vi "GoHome.vi"(4 "Home fail":refnum<vi>, 6 "HomeDone":refnum<vi>, 7 "Busy":refnum<vi>, 8 "error in (no error)":errorcluster, 11 "QuickSilver in":refnum<class "QuickSilver.lvclass">) -> (0 "error out":errorcluster, 2 "String":string, 3 "QuickSilver out":refnum<class "QuickSilver.lvclass">)   [LabVIEW 2012, in "QuickSilver.lvclass"]
uses:
  QuickSilver.lvclass
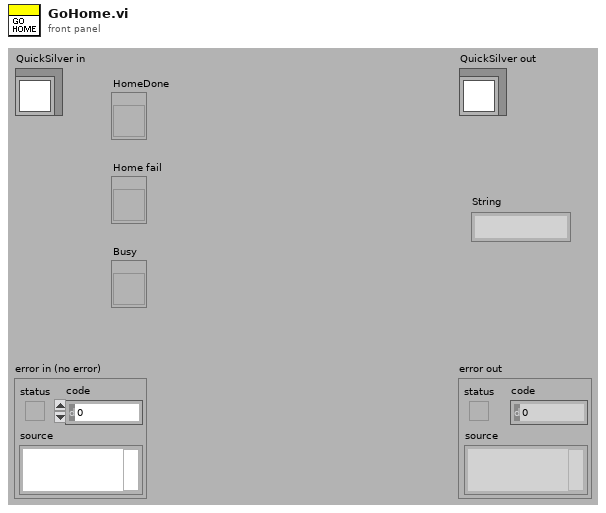
[diagram p1: front panel]
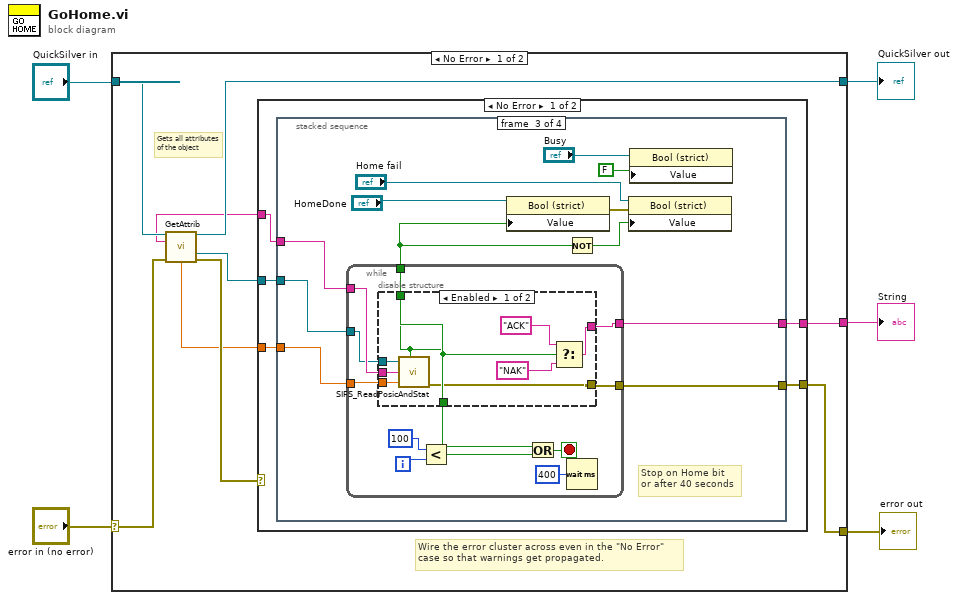
[diagram p0: block diagram]
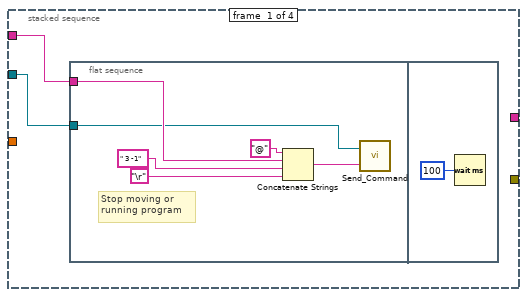
[diagram p2: hidden frame]
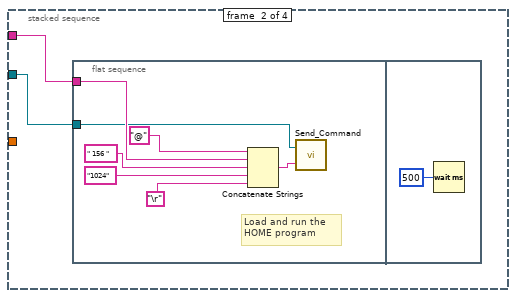
[diagram p3: hidden frame]
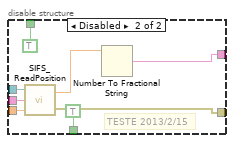
[diagram p4: hidden frame]
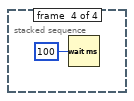
[diagram p5: hidden frame]
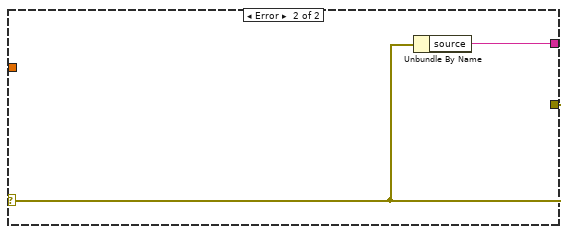
[diagram p6: hidden frame]
diagram:
  n1 = case shown="No Error" "error in (no error)" {
    selector: "error in (no error)" -> [w11 w82]
    tunnel: [w13 w82] -> w3
    tunnel: [w10 w81] -> w1
    tunnel: "QuickSilver in" -> [w12 w81]
    tunnel: [w14 _] -> w2
    frame No Error {
      # "Gets all attributes \nof the object"
      # "Wire the error cluster across even in the \"No Error\"\ncase so that warnings get propagated."
      n2 = call "GetAttrib.vi"("QuickSilver in"=w12, "error in (no error)"=w11) -> ("QuickSilver out"=w10:refnum<class "QuickSilver.lvclass">, "Mec ID"=w8:string, "VISA Mec"=w7:refnum<visa-resource-name>, "Mec Factor"=w6:dbl, "error out"=w9:errorcluster)  [unwired: 1 in, 8 out]
      n3 = case shown="No Error" w9 {
        selector: w9 -> [_ w80]
        tunnel: [w19 w79] -> w14
        tunnel: [w18 w80] -> w13
        tunnel: w8 -> [w17 _]
        tunnel: w7 -> [w16 _]
        tunnel: w6 -> [w15 _]
        frame No Error {
          n4 = stacked-sequence {
            tunnel: w17 -> [w21 w30 w49 _]
            tunnel: w16 -> [w20 w29 w50 _]
            tunnel: w15 -> [_ _ w48 _]
            tunnel: [_ _ w47 _] -> w18
            tunnel: [_ _ w46 _] -> w19
            frame #0 {
              n5 = flat-sequence {
                tunnel: w21 -> [w27]
                tunnel: w20 -> [w22]
                frame #0 {
                  # "Stop moving or\nrunning program"
                  n6 = Concatenate Strings("@", w27, " 3 -1", "\r") -> (w26:string)
                  n7 = call "Send_Command.vi"("write buffer"=w26, "VISA resource name"=w22) -> ()  [unwired: 1 out]
                }
                frame #1 {
                  n8 = Wait (ms)(milliseconds to wait=u32 100) -> ()  [unwired: 1 out]
                }
              }
            }
            frame #1 {
              n9 = flat-sequence {
                tunnel: w30 -> [w34]
                tunnel: w29 -> [w31]
                frame #0 {
                  # "Load and run the\nHOME program"
                  n10 = Concatenate Strings("@", w34, " 156 ", "1024" ("string"), "\r") -> (w37:string)
                  n11 = call "Send_Command.vi"("write buffer"=w37, "VISA resource name"=w31) -> ()  [unwired: 1 out]
                }
                frame #1 {
                  n12 = Wait (ms)(milliseconds to wait=u32 500) -> ()  [unwired: 1 out]
                }
              }
            }
            frame #2 {
              # "Stop on Home bit\nor after 40 seconds"
              n13 = while {
                tunnel: w50 -> [w54]
                tunnel: w49 -> [w56]
                tunnel: w48 -> [w55]
                tunnel: [w52] -> w47
                tunnel: [w51] -> w46
                tunnel: [w53] -> w43
                i -> [w59]
                stop <- w57 stop-if-true
                n14 = disable-structure shown="Enabled" {
                  disable-tunnel: w56 -> [w69 w76]
                  disable-tunnel: w55 -> [w68 w75]
                  disable-tunnel: [w67 w70] -> w52
                  disable-tunnel: w54 -> [w66 w77]
                  disable-tunnel: [w62 TRUE ("Home bit")] -> w53
                  disable-tunnel: [w63 w72] -> w51
                  disable-tunnel: [w62 TRUE ("Home bit")] -> _
                  frame Enabled {
                    n15 = call "SIFS_ReadPosicAndStat.vi"("VISA resource name"=w66, "ID"=w69, "FATOR"=w68) -> ("Home bit"=w62:bool, "error out"=w67:errorcluster)  [unwired: 4 out]
                    n16 = Select(t="ACK", s=w62, f="NAK") -> (s? t:f=w63:string)
                  }
                  frame Disabled {
                    # "TESTE 2013/2/15"
                    n17 = call "SIFS_ReadPosition.vi"("FATOR"=w75, "ID"=w76, "VISA resource name"=w77) -> ("error out"=w70:errorcluster, "Position"=w73:dbl)
                    n18 = Number To Fractional String(number=w73) -> (F-format string=w72:string)  [unwired: 3 in]
                  }
                }
                n19 = Less?(x=100, y=w59) -> (x < y?=w60:bool)
                n20 = Or(x=w53, y=w60) -> (x .or. y?=w57:bool)
                n21 = Wait (ms)(milliseconds to wait=u32 400) -> ()  [unwired: 1 out]
              }
              n22 = property class="Bool (strict)"(reference="HomeDone", "Value"=w43) -> (error out=w41:errorcluster)  [unwired: 1 in, 1 out]
              n23 = Not(x=w43) -> (.not. x?=w42:bool)
              n24 = property class="Bool (strict)"(reference="Home fail", error in=w41, "Value"=w42) -> ()  [unwired: 2 out]
              n25 = property class="Bool (strict)"(reference="Busy", "Value"=FALSE) -> ()  [unwired: 1 in, 2 out]
            }
            frame #3 {
              n26 = Wait (ms)(milliseconds to wait=u32 100) -> ()  [unwired: 1 out]
            }
          }
        }
        frame Error {
          n27 = Unbundle By Name(w80) -> ("source"=w79:string)
        }
      }
    }
    frame Error {
    }
  }
  "error out" <- w3
  "QuickSilver out" <- w1
  "String" <- w2
